vi "Warn Deprecated (LIBSSH2_KNOWNHOST_KEY_SSHDSS).vi"(8 "error in (no error)":errorcluster, 10 "typemask":T1 items=["TYPE_PLAIN"=1, "TYPE_SHA1"=2, "TYPE_CUSTOM"=3, "KEYENC_RAW"=65536, "KEYENC_BASE64"=131072, "KEY_RSA1"=262144, "KEY_SSHRSA"=524288, "KEY_SSHDSS (deprecated)"=786432, "KEY_ECDSA_256"=1048576, "KEY_ECDSA_384"=1310720, "KEY_ECDSA_521"=1572864, "KEY_ED25519"=1835008, "KEY_UNKNOWN"=3932160]) -> (0 "error out":errorcluster)   [LabVIEW 2017, in "libssh2.lvlib"]
uses:
  libssh2.lvlib
  libssh2_knownhost_typemask.ctl
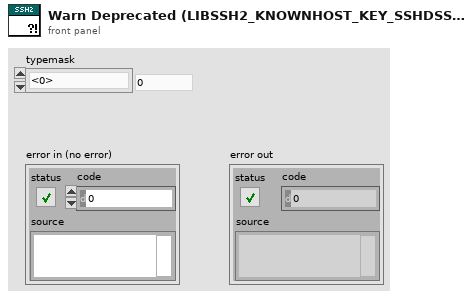
[diagram p1: front panel]
types:
  T1 = typedef "libssh2.lvlib/libssh2_knownhost_typemask.ctl" = i32
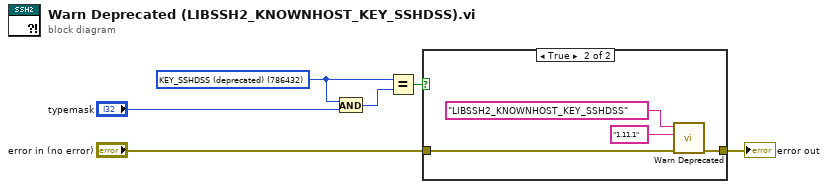
[diagram p0: block diagram]
diagram:
  w6 = T1 786432 items=["TYPE_PLAIN"=1, "TYPE_SHA1"=2, "TYPE_CUSTOM"=3, "KEYENC_RAW"=65536, "KEYENC_BASE64"=131072, "KEY_RSA1"=262144, "KEY_SSHRSA"=524288, "KEY_SSHDSS (deprecated)"=786432, "KEY_ECDSA_256"=1048576, "KEY_ECDSA_384"=1310720, "KEY_ECDSA_521"=1572864, "KEY_ED25519"=1835008, "KEY_UNKNOWN"=3932160] ("typemask")
  n1 = And(x=w6, y="typemask") -> (x .and. y?=w5:T1)
  n2 = Equal?(x=w6, y=w5) -> (x = y?=w4:bool)
  n3 = case shown="True" w4 {
    tunnel: "error in (no error)" -> [w7 w11]
    tunnel: [w7 w10] -> w2
    frame False {
    }
    frame True {
      n4 = call "Warn Deprecated.vi"("error in (no error)"=w11, "deprecated version"="1.11.1", "name"="LIBSSH2_KNOWNHOST_KEY_SSHDSS") -> ("error out"=w10:errorcluster)  [unwired: 8 in]
    }
  }
  "error out" <- w2
